vi "Trimmed white space.vi"() -> ()   [LabVIEW 2019]
panel:
  out "Length of the stripped string":i32
  out "Length of the input string":i32
  in  "Input string":string="           POMEGRANATE           "
  out "Trimmed string":string="POMEGRANATE"
  # "TRIMMED WHITE SPACE"
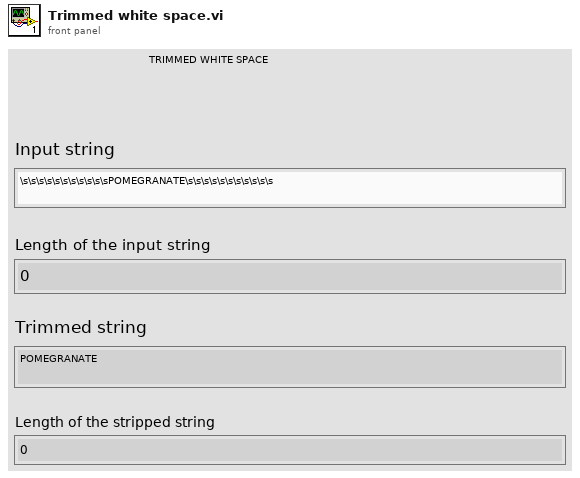
[diagram p1: front panel]
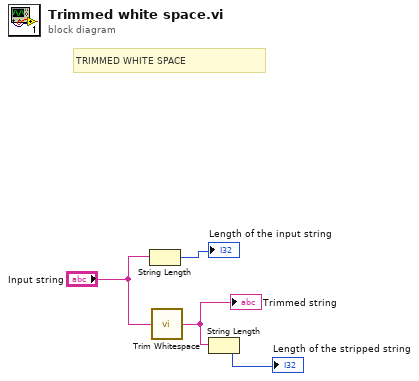
[diagram p0: block diagram]
diagram:
  # "TRIMMED WHITE SPACE"
  n1 = String Length(string="Input string") -> (length=→"Length of the input string":i32)
  n2 = call <vilib>:"Trim Whitespace.vi"("string"="Input string") -> ("trimmed string"=w2:string)  [unwired: 1 in]
  "Trimmed string" <- w2
  n3 = String Length(string=w2) -> (length=→"Length of the stripped string":i32)
